vi "API_Close.vi"(1 "VI Path":path, 2 "Argument List In":string[](array[string])) -> (0 "Argument List Out":string[](array[string]))   [LabVIEW 2011]
doc: "This VI opens a reference to the parent API VI via the \"VI Path\" parameter, then updates the \"Argument List\" with the values of all relevant front panel controls and indicators from the API VI."
panel:
  out "Error Out":errorcluster
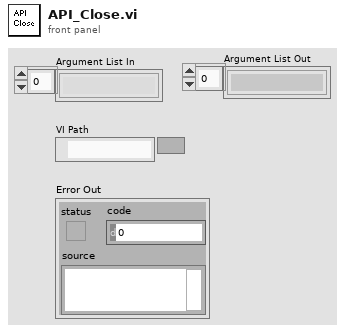
[diagram p1: front panel]
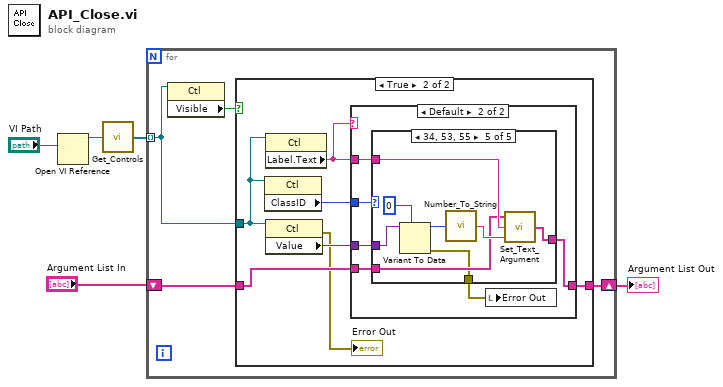
[diagram p0: block diagram]
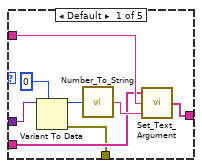
[diagram p4: hidden frame]
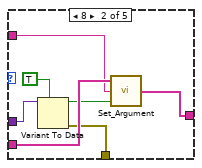
[diagram p5: hidden frame]
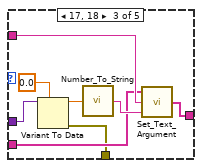
[diagram p6: hidden frame]
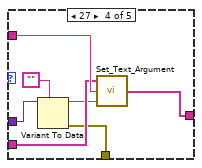
[diagram p7: hidden frame]
diagram:
  n1 = Open VI Reference(vi path="VI Path") -> (vi reference=w2:refnum<vi>)  [unwired: 5 in, 1 out]
  n2 = call "Get_Controls.vi"("VI Reference"=w2) -> ("Controls"=w1:refnum<vi>[])
  n3 = for {
    tunnel: w1 -> [w7] mode=indexing
    shift-right: [w8] -> w4
    shift-left: "Argument List In" -> [w9]
    n4 = property class="Ctl"(reference=w7) -> ("Visible"=w6:bool)  [unwired: 1 in, 2 out]
    n5 = case shown="True" w6 {
      tunnel: w9 -> [w10 w16]
      tunnel: [w10 w14] -> w8
      tunnel: w7 -> [_ w11]
      frame False {
      }
      frame True {
        n6 = property class="Ctl"(reference=w11) -> ("ClassID"=w17:u32)  [unwired: 1 in, 2 out]
        n7 = property class="Ctl"(reference=w11) -> ("Label.Text"=w12:string)  [unwired: 1 in, 2 out]
        n8 = property class="Ctl"(reference=w11) -> (error out=→"Error Out":errorcluster, "Value"=w15:variant)  [unwired: 1 in, 1 out]
        n9 = case shown="Default" w12 {
          tunnel: w17 -> [_ w24]
          tunnel: w16 -> [w18 w23]
          tunnel: w15 -> [_ w22]
          tunnel: w12 -> [_ w19]
          tunnel: [w18 w21] -> w14
          frame "Cancel", "OK" {
          }
          frame Default {
            n10 = case shown="34, 53, 55" w24 {
              tunnel: w23 -> [w30 w37 w42 w52 w60]
              tunnel: w22 -> [w28 w39 w47 w54 w58]
              tunnel: w19 -> [w31 w35 w43 w53 w61]
              tunnel: [w29 w34 w41 w51 w59] -> w21
              tunnel: [w25 w33 w40 w48 w55] -> w20
              frame Default {
                n11 = Variant To Data(type=0, Variant=w28) -> (data=w26:i32, error out=w25:errorcluster)  [unwired: 1 in]
                n12 = call "Number_To_String.vi"("Number"=w26) -> ("String"=w32:string)
                n13 = call "Set_Text_Argument.vi"("Text"=w32, "Argument"=w31, "Argument List In"=w30) -> ("Argument List Out"=w29:string[])
              }
              frame 8 {
                n14 = Variant To Data(type=TRUE, Variant=w39) -> (data=w36:bool, error out=w33:errorcluster)  [unwired: 1 in]
                n15 = call "Set_Argument.vi"("Enable"=w36, "Argument"=w35, "Argument List In"=w37) -> ("Argument List Out"=w34:string[])
              }
              frame 17, 18 {
                n16 = Variant To Data(type=0.0, Variant=w47) -> (data=w45:dbl, error out=w40:errorcluster)  [unwired: 1 in]
                n17 = call "Number_To_String.vi"("Number"=w45) -> ("String"=w44:string)
                n18 = call "Set_Text_Argument.vi"("Text"=w44, "Argument"=w43, "Argument List In"=w42) -> ("Argument List Out"=w41:string[])
              }
              frame 27 {
                n19 = Variant To Data(type="", Variant=w54) -> (data=w49:string, error out=w48:errorcluster)  [unwired: 1 in]
                n20 = call "Set_Text_Argument.vi"("Text"=w49, "Argument"=w53, "Argument List In"=w52) -> ("Argument List Out"=w51:string[])
              }
              frame 34, 53, 55 {
                n21 = Variant To Data(type=u16 0, Variant=w58) -> (data=w56:u16, error out=w55:errorcluster)  [unwired: 1 in]
                n22 = call "Number_To_String.vi"("Number"=w56) -> ("String"=w62:string)
                n23 = call "Set_Text_Argument.vi"("Text"=w62, "Argument"=w61, "Argument List In"=w60) -> ("Argument List Out"=w59:string[])
              }
            }
            n24 = local write "Error Out"(w20) -> ()
          }
        }
      }
    }
  }
  "Argument List Out" <- w4
